vi "MovingDateTransform.vi"(2 "INPUT":dbl[](array[numeric])) -> (0 "MOVEING COMMAND":string)   [LabVIEW 2014]
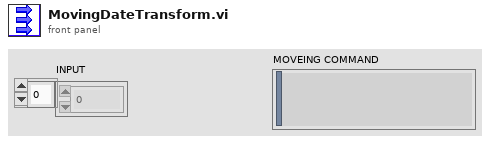
[diagram p1: front panel]
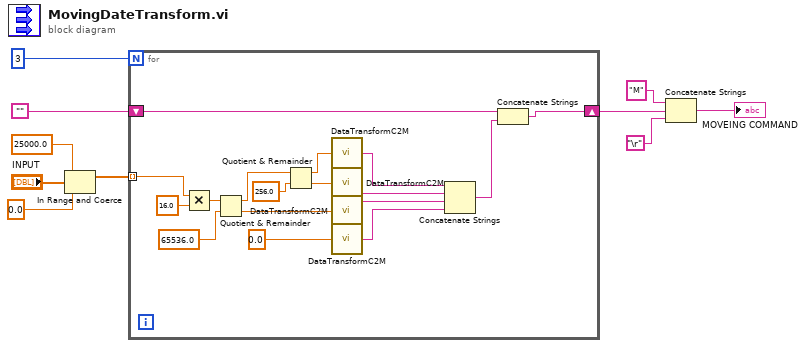
[diagram p0: block diagram]
diagram:
  n1 = In Range and Coerce ("判定范围并强制转换")(upper limit=25000.0 ("上限"), x="INPUT", lower limit=0.0 ("下限")) -> (coerced(x)=w3:dbl[])  [unwired: 1 out]
  n2 = for {
    N: 3 -> [_]
    tunnel: w3 -> [w14] mode=indexing
    shift-right: [w11] -> w8
    shift-left: "" -> [w13]
    n3 = Multiply(x=w14, y=16.0) -> (x*y=w24:dbl)
    n4 = Quotient & Remainder(x=w24, y=65536.0) -> (x-y*floor(x/y)=w26:dbl, floor(x/y)=w21:dbl)
    n5 = Quotient & Remainder(x=w26, y=256.0) -> (x-y*floor(x/y)=w19:dbl, floor(x/y)=w20:dbl)
    n6 = call "DataTransformC2M.vi"("input"=w19) -> ("output"=w18:string)
    n7 = call "DataTransformC2M.vi"("input"=w20) -> ("output"=w17:string)
    n8 = call "DataTransformC2M.vi"("input"=w21) -> ("output"=w16:string)
    n9 = call "DataTransformC2M.vi"("input"=0.0 ("number")) -> ("output"=w15:string)
    n10 = Concatenate Strings(w18, w17, w16, w15) -> (w12:string)
    n11 = Concatenate Strings(w13, w12) -> (w11:string)
  }
  n12 = Concatenate Strings("M" ("string"), w8, "\r") -> (→"MOVEING COMMAND":string)
